vi "Calibration Shooter.vi"() -> ()   [LabVIEW 2016]
uses:
  Framework/Robot Global Data.vi
  <vilib>/Rock Robotics/Network Tables/NT Read Number.vi
  <vilib>/Rock Robotics/SystemInterfaces/DIO/FPGA_DIOPWMChannel.ctl
  <vilib>/Rock Robotics/WPI/PWM/WPI_PWMDeadband.ctl
  <vilib>/Rock Robotics/WPI/MotorControl/WPI_MotorControlType.ctl
  <vilib>/Rock Robotics/WPI/MotorControl/WPI_MotorControlDeviceRef.ctl
  <vilib>/Rock Robotics/WPI/RobotDrive/WPI_RobotDriveDevRef.ctl
panel:
  in  "Distance from Wall (in)":dbl
  in  "Camera Height (in)":dbl
  in  "Shooter RPM":dbl
  in  "Next":bool
  out "Output":string
  in  "Cluster":cluster{"Start Time (ms)":u32, "Iterations":i32}
  in  "RobotDriveDevRef":T1
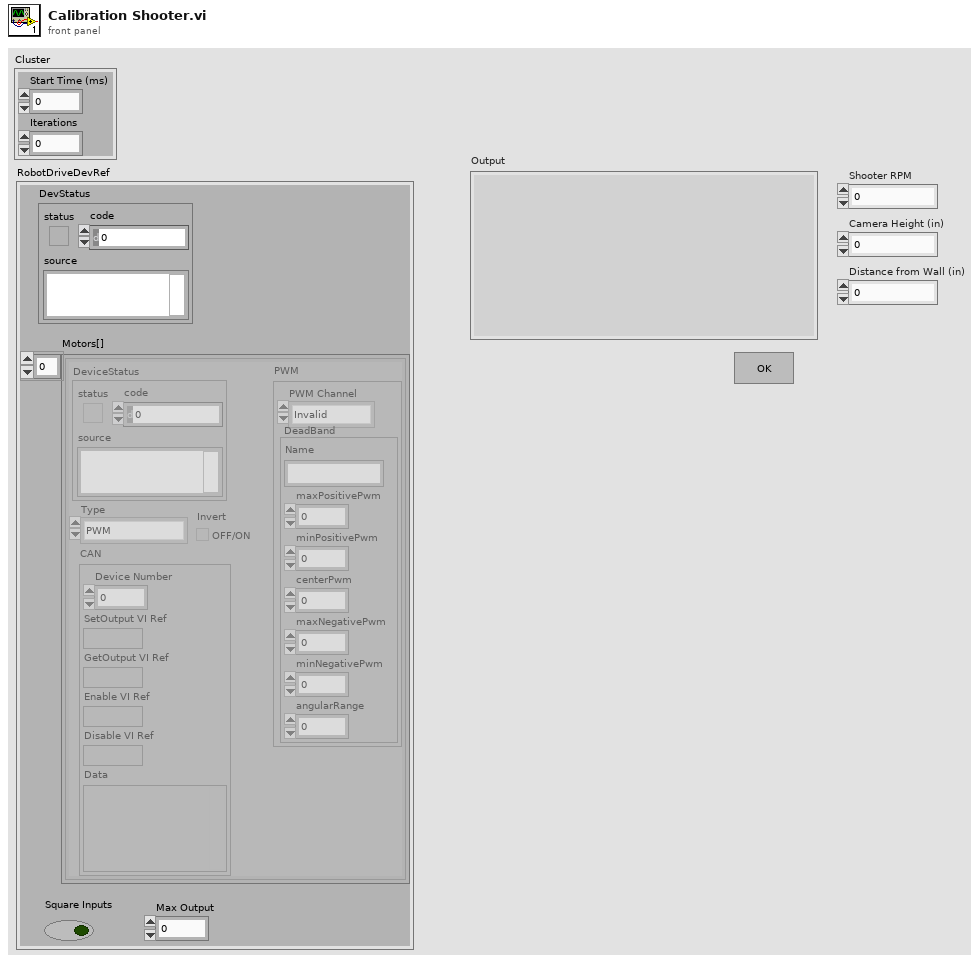
[diagram p1: front panel]
types:
  T1 = typedef "WPI_RobotDriveDevRef.ctl" = cluster{"DevStatus":errorcluster, "Motors[]":T2[], "Square Inputs":bool, "Max Output":dbl}
  T2 = typedef "WPI_MotorControlDeviceRef.ctl" = cluster{"DeviceStatus":errorcluster, "Type":T3, "PWM":cluster{"PWM Channel":T4, "DeadBand":T5}, "CAN":cluster{"Device Number":u8, "SetOutput VI Ref":variant, "GetOutput VI Ref":variant, "Enable VI Ref":variant, "Disable VI Ref":variant, "Data":variant}, "Invert":bool}
  T3 = typedef "WPI_MotorControlType.ctl" = enum16{"PWM", "CAN"}
  T4 = typedef "FPGA_DIOPWMChannel.ctl" = enum8{"PWM 0", "PWM 1", "PWM 2", "PWM 3", "PWM 4", "PWM 5", "PWM 6", "PWM 7", "PWM 8", "PWM 9", "PWM MXP 0", "PWM MXP 1", "PWM MXP 2", "PWM MXP 3", "PWM MXP 4", "PWM MXP 5", "PWM MXP 6", "PWM MXP 7", "PWM MXP 8", "PWM MXP 9", "Invalid"}
  T5 = typedef "WPI_PWMDeadband.ctl" = cluster{"Name":string, "maxPositivePwm":i32, "minPositivePwm":i32, "centerPwm":i32, "maxNegativePwm":i32, "minNegativePwm":i32, "angularRange":u16}
  T6 = typedef "NI_LVConfig.lvlib/Config Data RefNum.ctl" = refnum<k1>
  T7 = typedef "Dashboard Data.ctl" = cluster{"Drive PID - Low":T8, "Drive PID - High":T8, "Vision Settings":T9, "Robot Name":string, "Winch Out":dbl, "Winch In":dbl, "Shooter Settings":T10}
  T8 = typedef "PID Settings.ctl" = cluster{"D":dbl, "F":dbl, "RR":dbl, "IZ":dbl, "P":dbl, "I":dbl}
  T9 = typedef "Vision Data.ctl" = cluster{"LED Color":cluster{"Hue":cluster{dbl, dbl}, "Sat":cluster{dbl, dbl}, "Val":cluster{dbl, dbl}}, "Vision Line":dbl, "Vision Bottom Clip":dbl, "Gear Yaw Offset":dbl}
  T10 = typedef "Shooter Settings.ctl" = cluster{"Shooter PID":T8, "Instake Belt PID":T8, "Shooter Wheel RPM":dbl, "Instake Belt RPM":dbl, "Grinder Power":dbl, "Ramp Up Speed":dbl, "Cam Height":dbl, "Cam Angle":dbl, "Cam Yaw Offset":dbl}
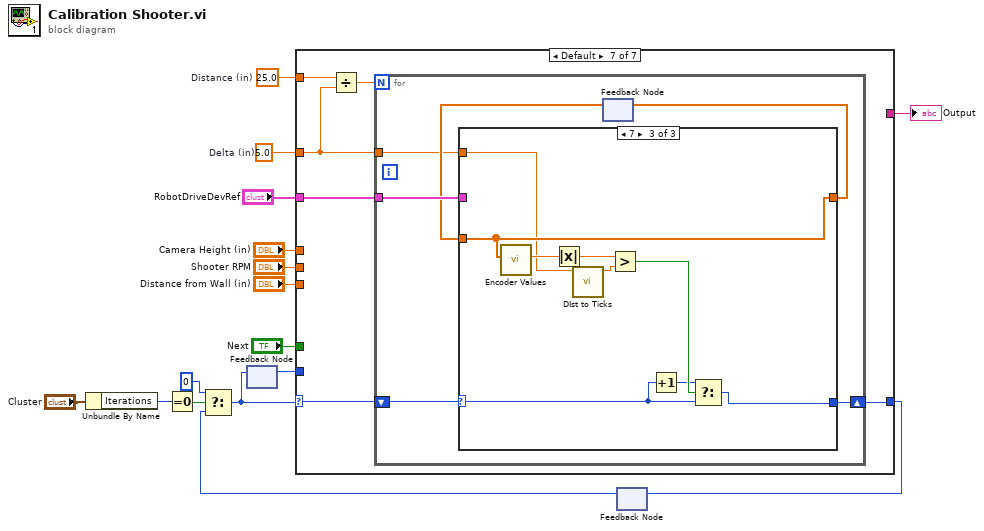
[diagram p0: block diagram]
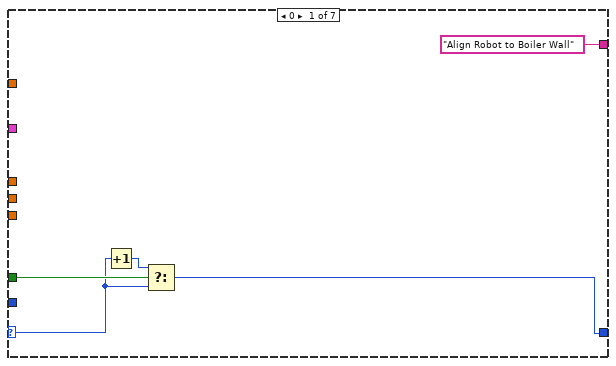
[diagram p2: hidden frame]
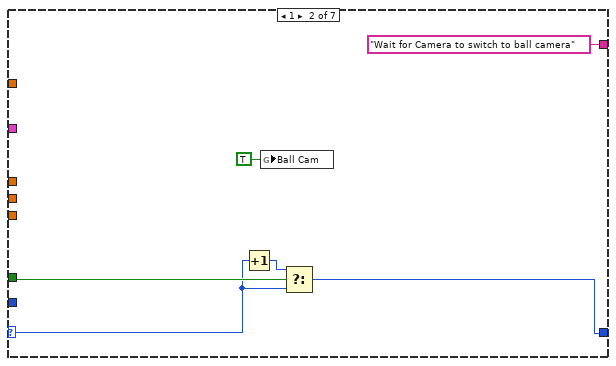
[diagram p3: hidden frame]
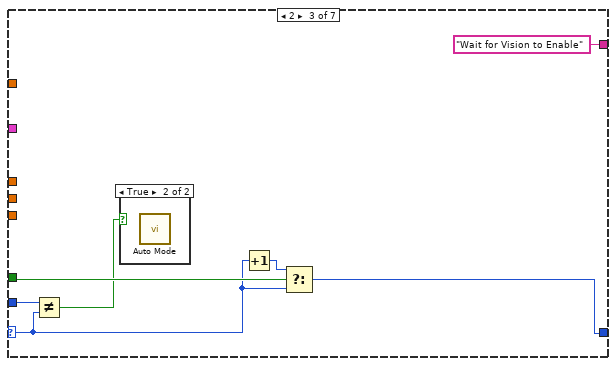
[diagram p4: hidden frame]
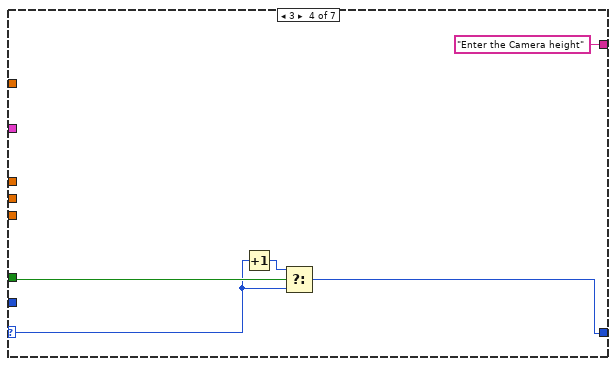
[diagram p6: hidden frame]
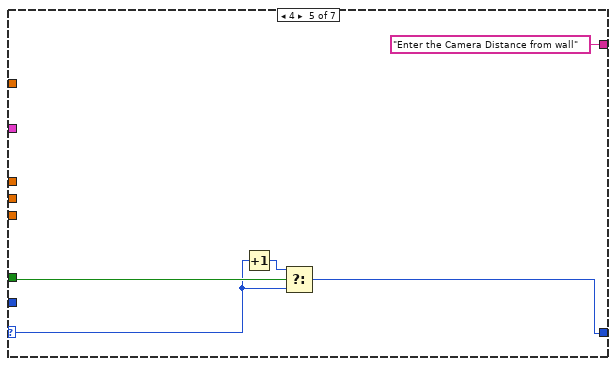
[diagram p7: hidden frame]
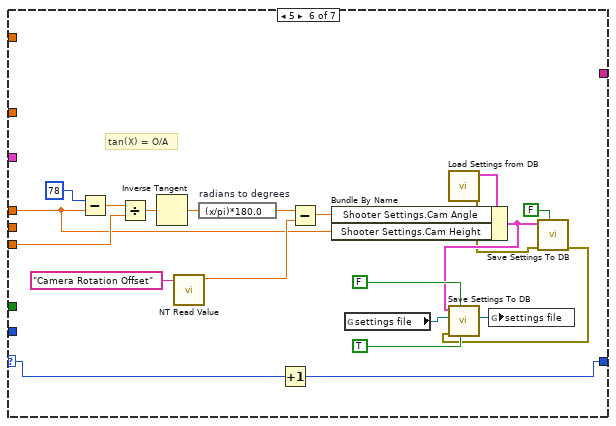
[diagram p8: hidden frame]
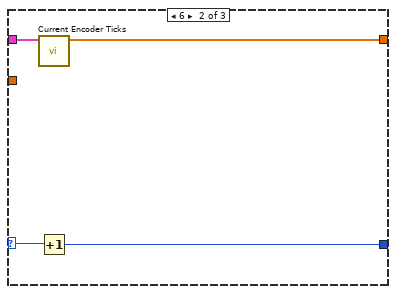
[diagram p10: hidden frame]
diagram:
  w5 = 25.0  # Distance (in)
  w6 = 5.0  # Delta (in)
  n1 = Unbundle By Name("Cluster") -> ("Iterations"=w15:i32)
  n2 = Equal To 0?(x=w15) -> (x = 0?=w14:bool)
  n3 = feedback #1() -> (w7:i32)  [unwired: 1 in]
  n4 = feedback #2() -> (w11:i32)  [unwired: 1 in]
  n5 = Select(t=0, s=w14, f=w11) -> (s? t:f=w8:i32)
  n6 = feedback-in #1(w8) -> ()
  n7 = case shown="Default" w8 {
    selector: w8 -> [w17 w23 w29 w35 w40 w46 w68]
    tunnel: [w19 w24 w31 w36 w41 w45 w66] -> w12
    tunnel: ["Align Robot to Boiler Wall" ("Output") "Wait for Camera to switch to ball camera" ("Output") "Wait for Vision to Enable" ("Output") "Enter the Camera height" ("Output") "Enter the Camera Distance from wall" ("Output") _ _] -> w10
    tunnel: "Next" -> [w20 w25 w32 w37 w42 _ _]
    tunnel: w7 -> [_ _ w30 _ _ _ _]
    tunnel: w6 -> [_ _ _ _ _ _ w69]
    tunnel: w5 -> [_ _ _ _ _ _ w71]
    tunnel: "RobotDriveDevRef" -> [_ _ _ _ _ _ w67]
    tunnel: "Camera Height (in)" -> [_ _ _ _ _ w55 _]
    tunnel: "Shooter RPM" -> [_ _ _ _ _ _ _]
    tunnel: "Distance from Wall (in)" -> [_ _ _ _ _ w63 _]
    frame 0 {
      n8 = Increment(x=w17) -> (x+1=w18:i32)
      n9 = Select(t=w18, s=w20, f=w17) -> (s? t:f=w19:i32)
    }
    frame 1 {
      n10 = Increment(x=w23) -> (x+1=w26:i32)
      n11 = global write "Robot Global Data.vi" "Ball Cam"(TRUE ("Ball Cam")) -> ()
      n12 = Select(t=w26, s=w25, f=w23) -> (s? t:f=w24:i32)
    }
    frame 2 {
      n13 = Not Equal?(x=w30, y=w29) -> (x != y?=w28:bool)
      n14 = case shown="True" w28 {
        frame False {
        }
        frame True {
          n15 = call "Auto Mode.vi"() -> ()  [unwired: 12 in]
        }
      }
      n16 = Increment(x=w29) -> (x+1=w33:i32)
      n17 = Select(t=w33, s=w32, f=w29) -> (s? t:f=w31:i32)
    }
    frame 3 {
      n18 = Increment(x=w35) -> (x+1=w38:i32)
      n19 = Select(t=w38, s=w37, f=w35) -> (s? t:f=w36:i32)
    }
    frame 4 {
      n20 = Increment(x=w40) -> (x+1=w43:i32)
      n21 = Select(t=w43, s=w42, f=w40) -> (s? t:f=w41:i32)
    }
    frame 5 {
      # "tan(X) = O/A"
      n22 = Subtract(x=78, y=w55) -> (x-y=w64:dbl)
      n23 = Divide(x=w64, y=w63) -> (x/y=w62:dbl)
      n24 = Inverse Tangent(1:w62) -> (0:w61:dbl)
      n25 = call-poly <vilib>:"NT Read Value.vi"("Name"="Camera Rotation Offset") -> ("Numeric"=w58:dbl)  [unwired: 9 in, 1 out]
      n26 = expression code="(x/pi)*180.0" "radians to degrees"(w61) -> (w60:dbl)
      n27 = Increment(x=w46) -> (x+1=w45:i32)
      n28 = Subtract(x=w60, y=w58) -> (x-y=w56:dbl)
      n29 = global read "Robot Global Data.vi" "settings file"() -> (w51:T6)
      n30 = call "Load Settings from DB.vi"() -> ("error out"=w47:errorcluster, "Dashboard Data (out)"=w57:T7)  [unwired: 10 in]
      n31 = Bundle By Name(cluster=w57, "Shooter Settings.Cam Angle"=w56, "Shooter Settings.Cam Height"=w55) -> (w49:T7)
      n32 = call "Save Settings To DB.vi"("Dashboard?"=FALSE, "error in"=w47, "Dashboard Data (in)"=w49) -> ("error out"=w48:errorcluster)  [unwired: 7 in, 1 out]
      n33 = call "Save Settings To DB.vi"("Save To File?"=TRUE, "Dashboard?"=FALSE, "error in"=w48, "save file (in)"=w51, "Dashboard Data (in)"=w49) -> ("save file (out)"=w50:T6)  [unwired: 5 in, 1 out]
      n34 = global write "Robot Global Data.vi" "settings file"(w50) -> ()
    }
    frame Default {
      n35 = Divide(x=w71, y=w69) -> (x/y=w70:dbl)
      n36 = for {
        N: w70 -> [_]
        tunnel: w69 -> [w73]
        tunnel: w67 -> [w76]
        shift-right: [w72] -> w66
        shift-left: w68 -> [w77]
        n37 = feedback #3() -> (w74:dbl[])  [unwired: 1 in]
        n38 = case shown="7" w77 {
          selector: w77 -> [_ w79 w83]
          tunnel: w73 -> [_ _ w86]
          tunnel: w76 -> [_ w81 _]
          tunnel: [_ w80 w87] -> w75
          tunnel: w74 -> [_ _ w87]
          tunnel: [_ w78 w84] -> w72
          frame 0, Default {
          }
          frame 6 {
            n39 = call "Current Encoder Ticks.vi"("RobotDriveDevRef"=w81) -> ("Array"=w80:dbl[])  [unwired: 10 in]
            n40 = Increment(x=w79) -> (x+1=w78:i32)
          }
          frame 7 {
            n41 = call "Encoder Values.vi"("Array"=w87) -> ("Position"=w88:dbl)  [unwired: 9 in, 1 out]
            n42 = Absolute Value(x=w88) -> (abs(x)=w89:dbl)
            n43 = call "DIst to Ticks.vi"("x"=w86) -> ("Numeric"=w90:dbl)  [unwired: 10 in]
            n44 = Greater?(x=w89, y=w90) -> (0:w85:bool)
            n45 = Increment(x=w83) -> (x+1=w82:i32)
            n46 = Select(t=w82, s=w85, f=w83) -> (s? t:f=w84:i32)
          }
        }
        n47 = feedback-in #3(w75) -> ()
      }
    }
  }
  "Output" <- w10
  n48 = feedback-in #2(w12) -> ()
